vi "OA Get Number Of User Modes.vi"(11 "puiNumberOfModes":u32) -> (2 "function return":u32, 3 "puiNumberOfModes out":u32)   [LabVIEW 2018, in "AndorSDK.lvlib"]
doc: "EXPNETTYPE unsigned int WINAPI OA_GetNumberOfUserModes(unsigned int * const puiNumberOfModes);"
uses:
  AndorSDK.lvlib
  ATMCD32D.dll
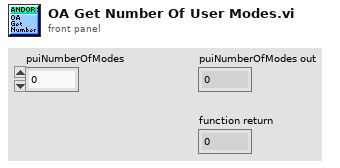
[diagram p1: front panel]
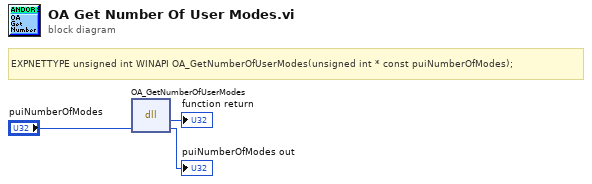
[diagram p0: block diagram]
diagram:
  # "EXPNETTYPE unsigned int WINAPI OA_GetNumberOfUserModes(unsigned int * const puiNumberOfModes);"
  n1 = dll-call lib="PTH2babs E\nPersönliches02 - Arbeit03-HiwijobsLabviewCodelibANDOR\tAndor SDK\nATMCD32D.*" fn="OA_GetNumberOfUserModes"("puiNumberOfModes"="puiNumberOfModes") -> (→"function return":u32, "puiNumberOfModes"=→"puiNumberOfModes out":u32)  [unwired: 3 in, 2 out]
